vi "Clear I2C Messages Table.vi"(5 "# TXNS IN TABLE Ref":refnum<vi>, 7 "I2C Table Ref":refnum<vi>, 8 "error in (no error)":errorcluster, 11 "Measurement UI Queue":refnum<queue>) -> (0 "error out":errorcluster)   [LabVIEW 2025, in "I2C Bus Monitor UI.lvlib"]
uses:
  I2C Bus Monitor UI.lvlib
  Table Buffer - Flush.vi
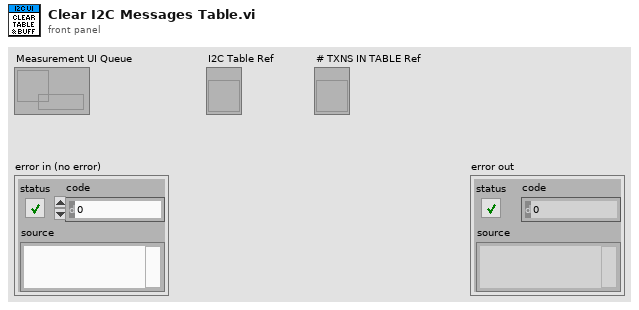
[diagram p1: front panel]
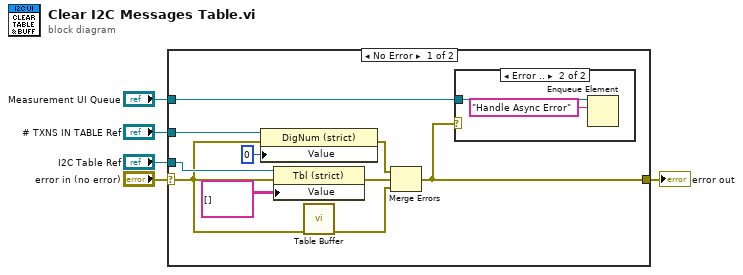
[diagram p0: block diagram]
diagram:
  n1 = case shown="No Error" "error in (no error)" {
    selector: "error in (no error)" -> [w12 w18]
    tunnel: "I2C Table Ref" -> [w15 _]
    tunnel: [w7 w18] -> w3
    tunnel: "# TXNS IN TABLE Ref" -> [w13 _]
    tunnel: "Measurement UI Queue" -> [w6 _]
    frame No Error {
      n2 = property on="Property Node" class="DigNum (strict)"(reference=w13, error in=w12, "Value"=0) -> (error out=w9:errorcluster)  [unwired: 1 out]
      n3 = property on="Property Node" class="Tbl (strict)"(reference=w15, error in=w12, "Value"=string[][] []) -> (error out=w10:errorcluster)  [unwired: 1 out]
      n4 = call-poly "Table Buffer.vi"("error in (no error)"=w12) -> ("error out"=w8:errorcluster)  [unwired: 10 in]
      n5 = Merge Errors(w9, w10, w8) -> (w7:errorcluster)
      n6 = case shown="Error .." w7 {
        tunnel: w6 -> [_ w17]
        frame No Error {
        }
        frame Error {
          n7 = Enqueue Element(queue=w17, element="Handle Async Error") -> ()  [unwired: 2 in, 3 out]
        }
      }
    }
    frame Error {
    }
  }
  "error out" <- w3
